vi "Polar Plot-Linear.vi"(6 "axis labels":string[](array[string])=["", "90", "180", "270"], 7 "top left point(0, 0)":cluster{"x":i16, "y":i16}, 8 "error in":errorcluster, 9 "dimensions (w,h)":cluster{"width":i16, "height":i16}, 10 "Polar Properties":T1={"polar attributes"={"maximum"=0.0, "minimum"=0.0, "clip to min"=FALSE, "log?(F)"=FALSE, "grid color"=6710886, "plot color"=16711680, "fmt and prec"={"format"=enum."Decimal", "precision"=0}, "visible section"=8}, "data array [mag, phase (deg)]"=[], "font"={"desired font(Application) "=enum."Application Font", "[user-specified font] "={"Font Name:"="", "Size"=0, "Strikeout?"=FALSE, "Italic?"=FALSE, "Underline?"=FALSE, "Outline?"=FALSE, "Shadow?"=FALSE, "Bold?"=FALSE}}, "Scale Polar plot"=0.2, "Size"=1} {"data array [mag, phase (deg)]"."phase" format="%0.2f"; "data array [mag, phase (deg)]"."magnitude" format="%0.2f"; "polar attributes"."minimum" format="%0.3f"; "polar attributes"."maximum" format="%0.3f"}, 11 "picture In":picture) -> (0 "error Out":errorcluster, 3 "picture out":picture)   [LabVIEW 2020]
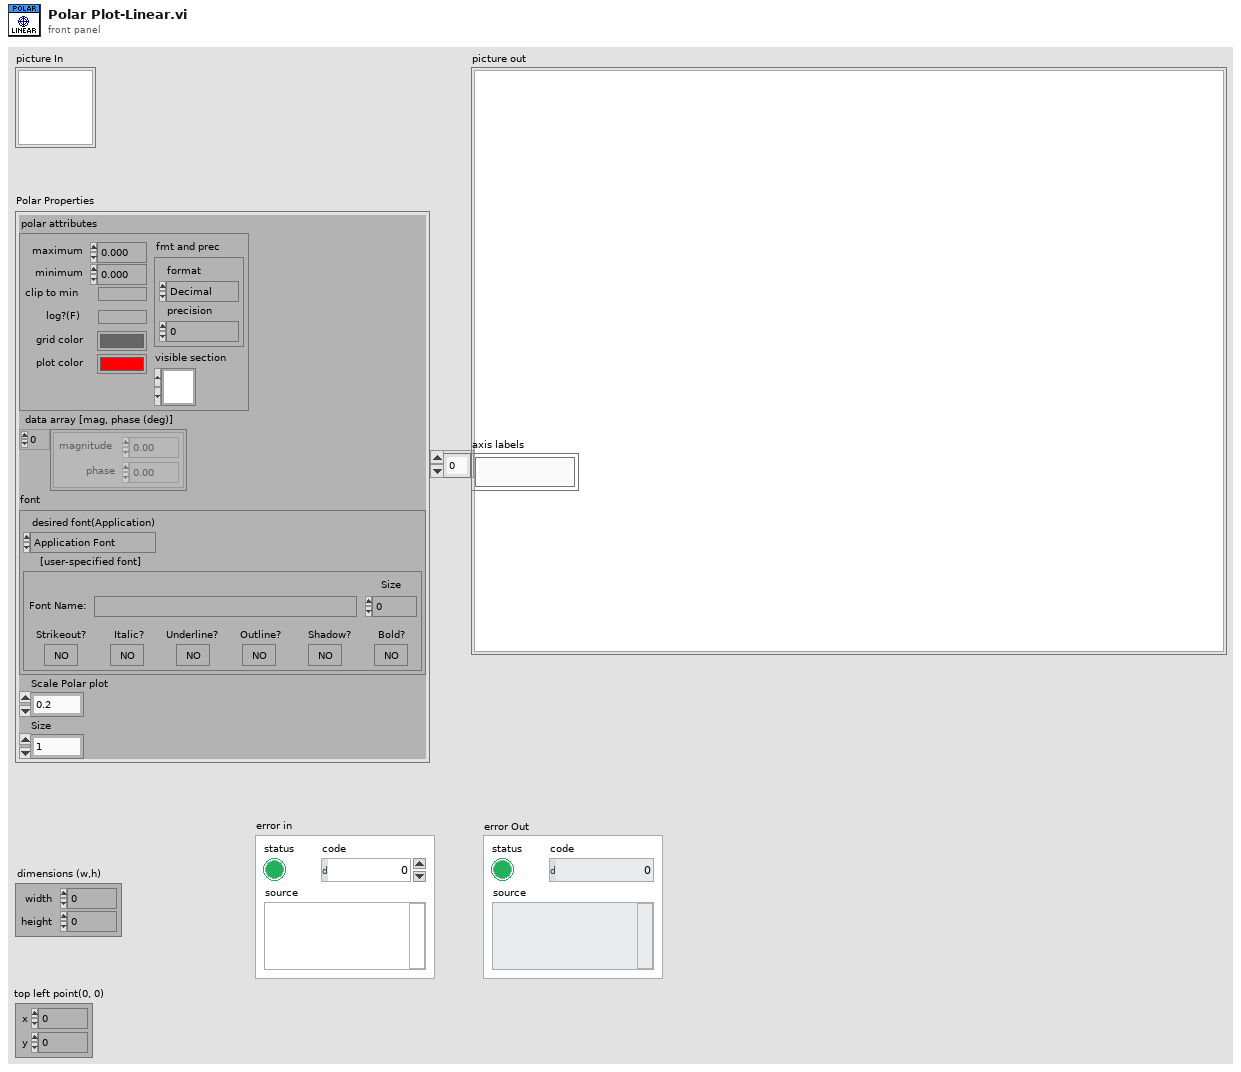
[diagram p1: front panel]
types:
  T1 = cluster{"polar attributes":cluster{"maximum":dbl, "minimum":dbl, "clip to min":bool, "log?(F)":bool, "grid color":u32, "plot color":u32, "fmt and prec":cluster{"format":enum8{"Decimal", "Scientific", "Engineering", "Binary", "Octal", "Hex"}, "precision":u8}, "visible section":u16}, "data array [mag, phase (deg)]":cluster{"magnitude":dbl, "phase":dbl}[], "font":cluster{"desired font(Application) ":enum16{"User-specified Font", "Application Font", "System Font", "Dialog Font"}, "[user-specified font] ":cluster{"Font Name:":string, "Size":i16, "Strikeout?":bool, "Italic?":bool, "Underline?":bool, "Outline?":bool, "Shadow?":bool, "Bold?":bool}}, "Scale Polar plot":dbl, "Size":u16}
  T2 = enum16{"User-specified Font", "Application Font", "System Font", "Dialog Font"}
  T3 = cluster{"Font Name:":string, "Size":i16, "Strikeout?":bool, "Italic?":bool, "Underline?":bool, "Outline?":bool, "Shadow?":bool, "Bold?":bool}
  T4 = cluster{"maximum":dbl, "minimum":dbl, "clip to min":bool, "log?(F)":bool, "grid color":u32, "plot color":u32, "fmt and prec":cluster{"format":enum8{"Decimal", "Scientific", "Engineering", "Binary", "Octal", "Hex"}, "precision":u8}, "visible section":u16}
  T5 = cluster{"left":i16, "top":i16, "right":i16, "bottom":i16}
  T6 = cluster{"pixel center":cluster{"x":i16, "y":i16}, "scale factors":cluster{"a":dbl, "b":dbl, "log?(F)":bool}, "grid color":u32, "start angle":dbl, "end angle":dbl, "tick length":i16, "pixel radius":i32}
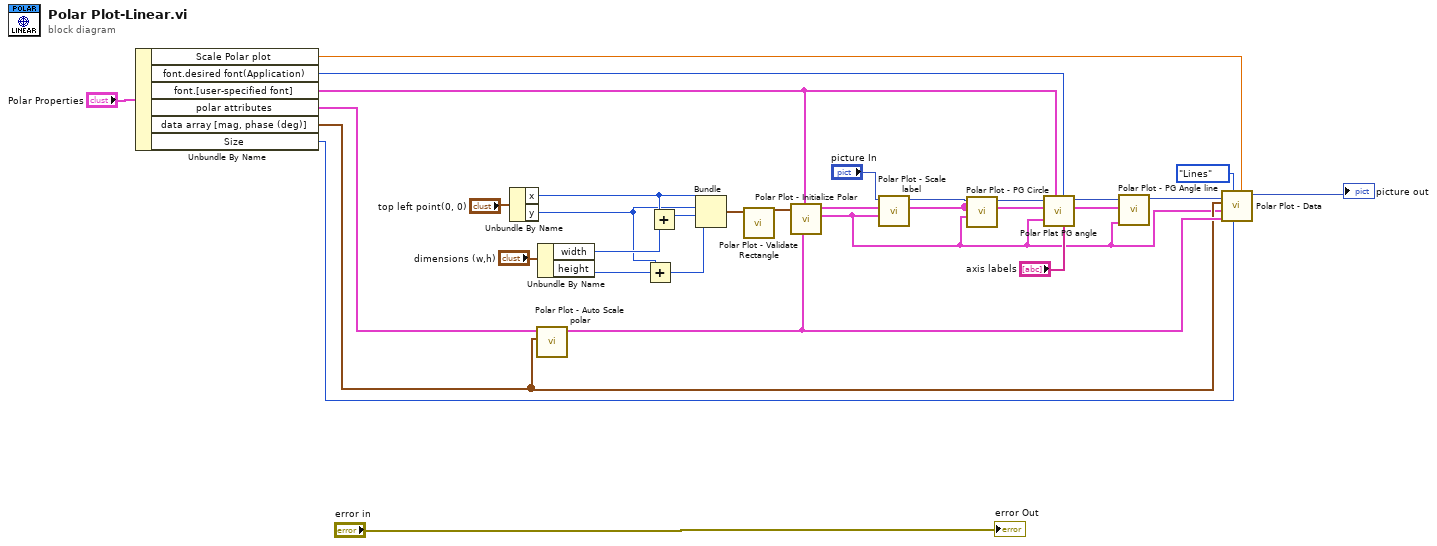
[diagram p0: block diagram]
diagram:
  n1 = Unbundle By Name("Polar Properties") -> ("Scale Polar plot"=w8:dbl, "font.desired font(Application)"=w17:T2, "font.[user-specified font]"=w18:T3, "polar attributes"=w9:T4, "data array [mag, phase (deg)]"=w10:cluster{"magnitude":dbl, "phase":dbl}[], "Size"=w7:u16)
  n2 = Unbundle By Name("top left point(0, 0)") -> ("x"=w25:i16, "y"=w24:i16)
  n3 = call "Polar Plot - Auto Scale polar.vi"("data"=w10, "polar attributes"=w9) -> ("polar attributes"=w15:T4)  [unwired: 9 in]
  n4 = Unbundle By Name("dimensions (w,h)") -> ("width"=w27:i16, "height"=w26:i16)
  n5 = Add(x=w24, y=w26) -> (x+y=w22:i16)
  n6 = Add(x=w25, y=w27) -> (x+y=w23:i16)
  n7 = Bundle("x"=w25, "y"=w24, w23, w22) -> (w21:cluster{"x":i16, "y":i16, i16, i16})  [unwired: 1 in]
  n8 = call "Polar Plot - Validate Rectangle.vi"("rect"=w21) -> ("valid rect"=w20:T5)  [unwired: 10 in]
  n9 = call "Polar Plot - Initialize Polar.vi"("polar attributes"=w15, "[user-specified font]"=w18, "rect"=w20) -> ("grid measurements"=w1:T6, "scale specs"=w2:cluster{"coordinate":i16, "label":string}[])  [unwired: 7 in]
  n10 = call "Polar Plot - Scale label.vi"("grid measurements"=w1, "scale specs"=w2, "picture"="picture In") -> ("new picture"=w4:picture)  [unwired: 8 in]
  n11 = call "Polar Plot - PG Circle.vi"("grid measurements"=w1, "decade specs"=w2, "picture"=w4) -> ("new picture"=w3:picture)  [unwired: 8 in]
  n12 = call "Polar Plat PG angle.vi"("axis labels"="axis labels", "desired font(Application)"=w17, "grid measurements"=w1, "[user-specified font]"=w18, "picture  in"=w3) -> ("picture  out"=w16:picture)  [unwired: 6 in]
  n13 = call "Polar Plot - PG Angle line.vi"("grid measurements"=w1, "decade specs"=w2, "picture"=w16) -> ("new picture"=w14:picture)  [unwired: 8 in]
  n14 = call "Polar Plot - Data.vi"("Scale Polar plot"=w8, "Size"=w7, "Lines/Points"=enum16{"Lines", "Points"}."Lines", "polar attributes"=w15, "grid measurements"=w1, "data array [mag, phase (deg)]"=w10, "new picture in"=w14) -> ("new picture out"=→"picture out":picture)  [unwired: 3 in, 1 out]
  "error Out" <- "error in"
